vi "buffer size set.vi"(10 "bytes per plot":ext, 11 "max number of sampels on the memory":ext) -> (3 "buffer size":ext)   [LabVIEW 2021]
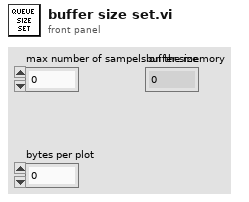
[diagram p1: front panel]
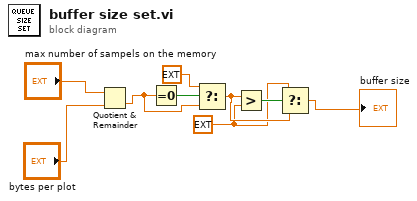
[diagram p0: block diagram]
diagram:
  w2 = ext 3.0 ("y")
  n1 = Quotient & Remainder(x="max number of sampels on the memory", y="bytes per plot") -> (floor(x/y)=w6:ext)  [unwired: 1 out]
  n2 = Equal To 0?(x=w6) -> (x = 0?=w5:bool)
  n3 = Select(t=ext 1.0, s=w5, f=w6) -> (s? t:f=w3:ext)
  n4 = Greater?(x=w3, y=w2) -> (0:w4:bool)
  n5 = Select(t=w2, s=w4, f=w3) -> (s? t:f=→"buffer size":ext)
